vi "indexArgVarArrInSecVar.vi"(9 "*sec":string, 11 "*sec+arg* 2D":string[][](array[string])) -> (3 "argVarArrIn*sec":string[](array[string]))   [LabVIEW 2010]
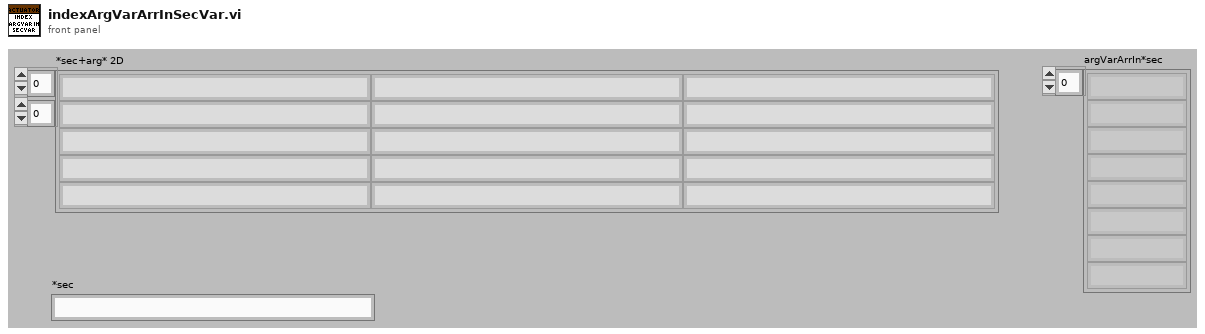
[diagram p1: front panel]
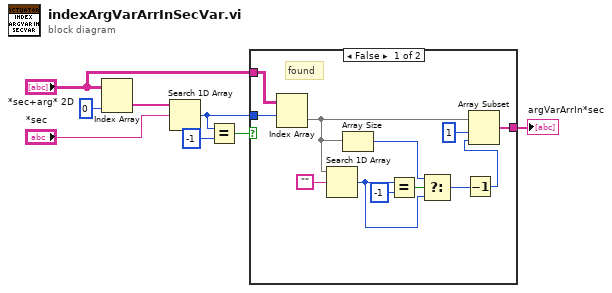
[diagram p0: block diagram]
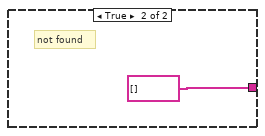
[diagram p2: hidden frame]
diagram:
  n1 = Index Array(array="*sec+arg* 2D", index (col)=0 ("disabled index (col)")) -> (element=w7:string[])  [unwired: 1 in]
  n2 = Search 1D Array(1D array=w7, element="*sec") -> (index of element=w3:i32)  [unwired: 1 in]
  n3 = Equal?(x=w3, y=-1) -> (x = y?=w4:bool)
  n4 = case shown="False" w4 {
    tunnel: w3 -> [w20 _]
    tunnel: "*sec+arg* 2D" -> [w19 _]
    tunnel: [w16 string[] []] -> w1
    frame False {
      # "found"
      n5 = Index Array(array=w19, index (row)=w20) -> (element=w13:string[])  [unwired: 1 in]
      n6 = Search 1D Array(1D array=w13, element="") -> (index of element=w11:i32)  [unwired: 1 in]
      n7 = Array Size(array=w13) -> (size(s)=w12:i32)
      n8 = Equal?(x=w11, y=-1) -> (x = y?=w14:bool)
      n9 = Select(t=w12, s=w14, f=w11) -> (s? t:f=w10:i32)
      n10 = Decrement(x=w10) -> (x-1=w9:i32)
      n11 = Array Subset(array=w13, index=1, length=w9) -> (w16:string[])
    }
    frame True {
      # "not found"
    }
  }
  "argVarArrIn*sec" <- w1
